vi "WSVCAP SHL FPGA LL Procedure I2C - Send Address Byte.vi"(0 "Procedure Step":T1, 1 "Wait Ticks Remaining":u32, 5 "I2C Wait Ticks":u32, 7 "Write Bits Remaining":u8, 9 "Write Byte":u8, 11 "error in (no error)":errorcluster, 13 "Socket Mask":u64 format="%012x", 14 "UUT Set (0/1)":u8) -> (3 "Wait Ticks Remaining Out":u32, 4 "Procedure Step Out":T1, 8 "Write Bits Remaining Out":u8, 10 "Finished":bool, 15 "error out":errorcluster)   [LabVIEW 2017]
uses:
  Type Defs/WSVCAP SHL Procedure Step Enum.ctl
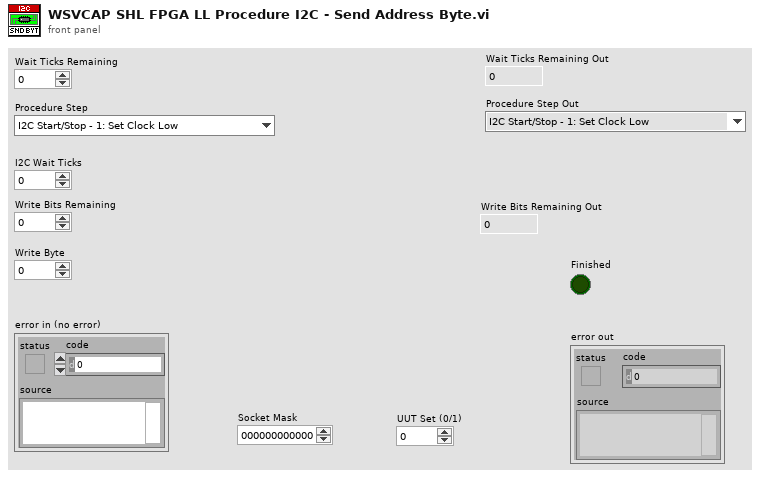
[diagram p1: front panel]
types:
  T1 = typedef "WSVCAP SHL Procedure Step Enum.ctl" = enum16{"I2C Start/Stop - 1: Set Clock Low", "I2C Start/Stop - 2: Wait", "I2C Start/Stop - 3: Set Data I", "I2C Start/Stop - 4: Wait", "I2C Start/Stop - 5: Set Clock High", "I2C Start/Stop - 6: Wait", "I2C Start/Stop - 7: Set Data II", "I2C Start/Stop - 8: Wait", "I2C Start/Stop - 9: Set Clock Low", "I2C Start/Stop - 10: Wait", "I2C Read ACK - 1: Set Clock High", "I2C Read ACK - 2: Wait", "I2C Read ACK - 3: Read ACK Bit", "I2C Read ACK - 4: Wait", "I2C Read ACK - 5: Set Clock Low", "I2C Read ACK - 6: Wait", "I2C Write ACK - 1: Write ACK Bit", "I2C Write ACK - 2: Wait", "I2C Write ACK - 3: Set Clock High", "I2C Write ACK - 4: Wait", "I2C Write ACK - 5: Set Clock Low", "I2C Write ACK - 6: Wait", "I2C Write ACK - 7: Set Data Low", "I2C Send Add - 1: Reset Bits Remaining", "I2C Send Add - 2: Set Data Bit", "I2C Send Add - 3: Wait", "I2C Send Add - 4: Set Clock High", "I2C Send Add - 5: Wait", "I2C Send Add - 6: Set Clock Low", "I2C Send Add - 7: Wait", "I2C Send Add - 8: Check Bits Remaining", "I2C Send Data - 1: Reset Bits Remaining", "I2C Send Data - 2: Load Write Bit from FIFO", "I2C Send Data - 3: Set Data Bit", "I2C Send Data - 4: Wait", "I2C Send Data - 5: Set Clock High", "I2C Send Data - 6: Wait", "I2C Send Data - 7: Set Clock Low", "I2C Send Data - 8: Wait", "I2C Send Data - 9: Check Bits Remaining", "I2C Receive Data - 1: Reset Bits Remaining", "I2C Receive Data - 2: Wait", "I2C Receive Data - 3: Set Clock High", "I2C Receive Data - 4: Wait", "I2C Receive Data - 5: Read Data Bit", "I2C Receive Data - 6: Wait", "I2C Receive Data - 7: Set Clock Low", "I2C Receive Data - 8: Wait", "I2C Receive Data - 9: Check Bits Remaining", "RFFE Send SSC - 1:Set Low", "RFFE Send SSC - 2:Wait", "RFFE Send SSC - 3:Set SDA High", "RFFE Send SSC - 4:Wait", "RFFE Send SSC - 5:Set SDA Low", "RFFE Send SSC - 6:Wait", "RFFE Send Data - 1:Set SCL High", "RFFE Send Data - 2:Wait", "RFFE Send Data - 3:Set SCL Low", "RFFE Send Data - 4:Wait", "RFFE Send Data - 5:Set SCL High (P)", "RFFE Send Data - 6:Wait", "RFFE Send Data - 7:Set SCL Low (P)", "RFFE Send Data - 8:Wait", "RFFE Send Data - 9:Set SCL High (BP)", "RFFE Send Data - 10:Wait", "RFFE Send Data - 11:Set SCL Low (BP)", "RFFE Send Data - 12:Wait", "RFFE Receive Data - 1:Set SCL High", "RFFE Receive Data - 2:Wait", "RFFE Receive Data - 3:Set SCL Low", "RFFE Receive Data - 4:Wait", "RFFE Receive Data - 5:Set SCL High (BP)", "RFFE Receive Data - 6:Wait", "RFFE Receive Data - 7:Set SCL Low (BP)", "RFFE Receive Data - 8:Wait", "RFFE Wait CMD Delay - 1:Wait", "RFFE Clear Lines - 1:Clear", "SRL Write Data - 1:Set SYNC High", "SRL Write Data - 2:Wait SYNC Delay", "SRL Write Data - 3:Set SYNC Low", "SRL Write Data - 4:Set SCLK High", "SRL Write Data - 5:Wait", "SRL Write Data - 6:Set SCLK Low", "SRL Write Data - 7:Wait", "SRL Write Data - 8:Set SYNC High", "SRL Wait CMD Delay - 1:Wait", "SRL Clear Lines - 1:Clear"}
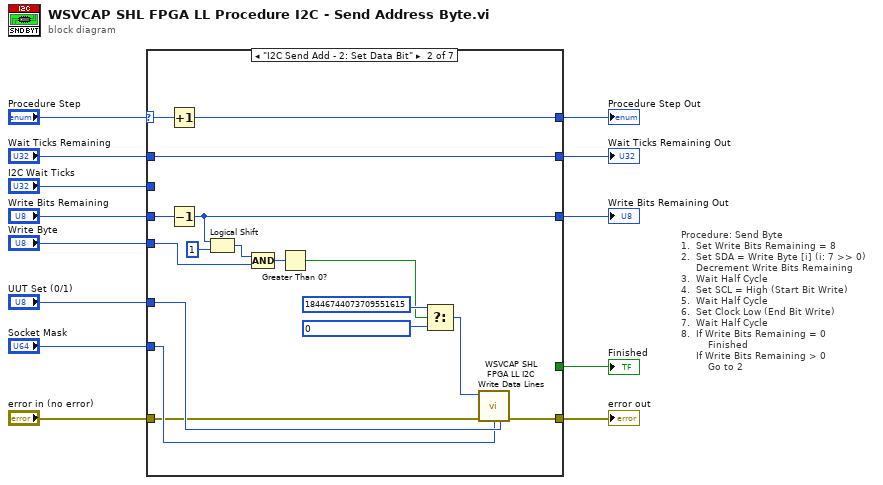
[diagram p0: block diagram]
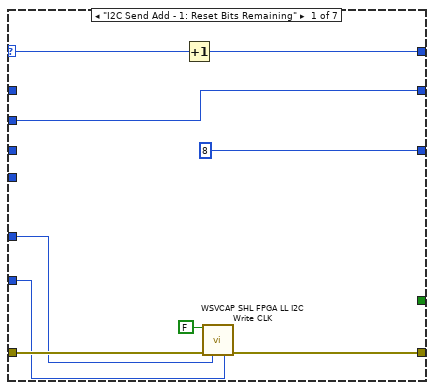
[diagram p2: hidden frame]
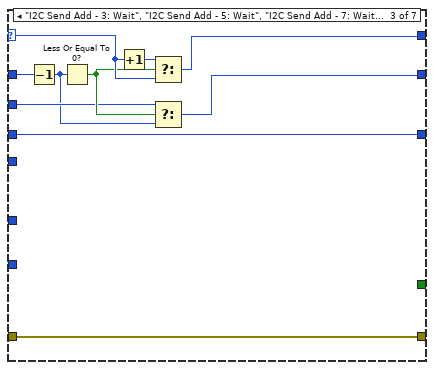
[diagram p3: hidden frame]
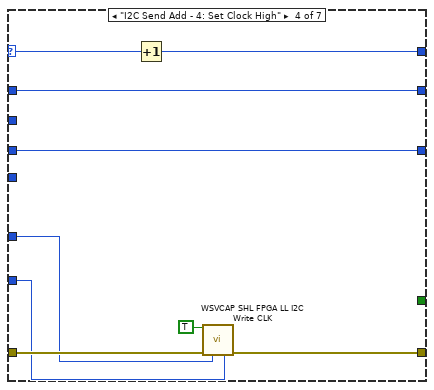
[diagram p4: hidden frame]
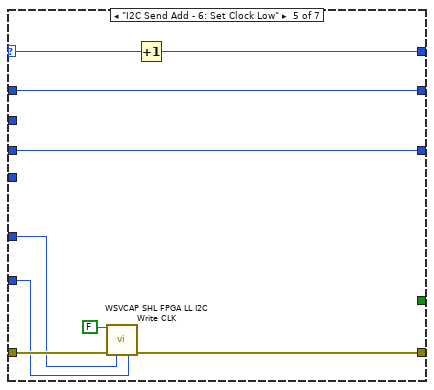
[diagram p5: hidden frame]
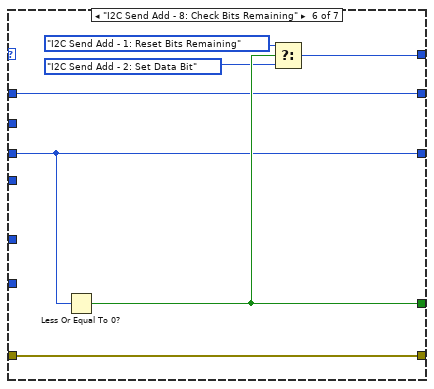
[diagram p6: hidden frame]
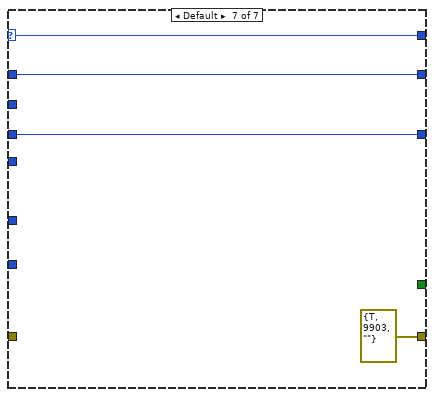
[diagram p7: hidden frame]
diagram:
  # "Procedure: Send Byte\n1.  Set Write Bits Remaining = 8\n2.  Set SDA = Write Byte [i] (i: 7 >> 0)\n     Decrement Write Bits Remaining\n3.  Wait Half Cycle\n4.  Set SCL = High (Start Bit Write)\n5.  Wait Half Cycle\n6.  Set Clock Low (End Bit Write)\n7.  Wait Half Cycle\n8.  If Write Bits Remaining = 0\n         Finished\n     If Write Bits Remaining > 0\n         Go to 2"
  n1 = case shown="\"I2C Send Add - 2: Set Data Bit\"" "Procedure Step" {
    selector: "Procedure Step" -> [w19 w39 w48 w56 w64 _ w77]
    tunnel: [w21 w23 w46 w57 w66 w74 errorcluster {"status"=TRUE, "code"=9903, "source"=""} ("error IO")] -> w12
    tunnel: "error in (no error)" -> [w22 w24 w46 w58 w67 w74 _]
    tunnel: "Wait Ticks Remaining" -> [_ w34 w49 w52 w61 w68 w76]
    tunnel: "I2C Wait Ticks" -> [w15 _ w44 _ _ _ _]
    tunnel: "Write Bits Remaining" -> [_ w37 w40 w51 w60 w69 w75]
    tunnel: "Write Byte" -> [_ w36 _ _ _ _ _]
    tunnel: [_ _ _ _ _ w73 _] -> w11
    tunnel: "Socket Mask" -> [w18 w25 _ w54 w63 _ _]
    tunnel: [w17 w35 w42 w53 w62 w70 w77] -> w4
    tunnel: [w15 w34 w41 w52 w61 w68 w76] -> w3
    tunnel: [u8 8 ("Write Bits Remaining") w33 w40 w51 w60 w69 w75] -> w2
    tunnel: "UUT Set (0/1)" -> [w14 w26 _ w50 w59 _ _]
    frame "I2C Send Add - 1: Reset Bits Remaining" {
      n2 = Increment(x=w19) -> (x+1=w17:T1)
      n3 = call "WSVCAP SHL FPGA LL I2C Write CLK.vi"("Bit In"=FALSE, "error in (no error)"=w22, "UUT Set (0/1 (Legacy)"=w14, "Socket Mask"=w18) -> ("error out"=w21:errorcluster)  [unwired: 11 in]
    }
    frame "I2C Send Add - 2: Set Data Bit" {
      n4 = Increment(x=w39) -> (x+1=w35:T1)
      n5 = Decrement(x=w37) -> (x-1=w33:u8)
      n6 = Logical Shift(y=w33, x=u8 1) -> (x << y=w31:u8)
      n7 = Compound Arithmetic op=AND(w31, w36) -> (w38:u8)
      n8 = Greater Than 0?(x=w38) -> (x > 0?=w27:bool)
      n9 = Select(t=u64 18446744073709551615 ("Write Bit (U64)"), s=w27, f=u64 0 ("Write Bit (U64)")) -> (s? t:f=w28:u64)
      n10 = call "WSVCAP SHL FPGA LL I2C Write Data Lines.vi"("Write Bit (U64)"=w28, "error in (no error)"=w24, "Socket Mask"=w25, "UUT Set (0/1) (Legacy)"=w26) -> ("error out"=w23:errorcluster)  [unwired: 11 in]
    }
    frame "I2C Send Add - 3: Wait", "I2C Send Add - 5: Wait", "I2C Send Add - 7: Wait" {
      n11 = Decrement(x=w49) -> (x-1=w43:u32)
      n12 = Less Or Equal To 0?(x=w43) -> (x <= 0?=w45:bool)
      n13 = Increment(x=w48) -> (x+1=w47:T1)
      n14 = Select(t=w47, s=w45, f=w48) -> (s? t:f=w42:T1)
      n15 = Select(t=w44, s=w45, f=w43) -> (s? t:f=w41:u32)
    }
    frame "I2C Send Add - 4: Set Clock High" {
      n16 = Increment(x=w56) -> (x+1=w53:T1)
      n17 = call "WSVCAP SHL FPGA LL I2C Write CLK.vi"("Bit In"=TRUE, "error in (no error)"=w58, "UUT Set (0/1 (Legacy)"=w50, "Socket Mask"=w54) -> ("error out"=w57:errorcluster)  [unwired: 11 in]
    }
    frame "I2C Send Add - 6: Set Clock Low" {
      n18 = call "WSVCAP SHL FPGA LL I2C Write CLK.vi"("Bit In"=FALSE, "error in (no error)"=w67, "UUT Set (0/1 (Legacy)"=w59, "Socket Mask"=w63) -> ("error out"=w66:errorcluster)  [unwired: 11 in]
      n19 = Increment(x=w64) -> (x+1=w62:T1)
    }
    frame "I2C Send Add - 8: Check Bits Remaining" {
      n20 = Less Or Equal To 0?(x=w69) -> (x <= 0?=w73:bool)
      n21 = Select(t=WSVCAP_SHL_Procedure_Step_Enum."I2C Send Add - 1: Reset Bits Remaining" ("Procedure Step"), s=w73, f=WSVCAP_SHL_Procedure_Step_Enum."I2C Send Add - 2: Set Data Bit" ("Procedure Step")) -> (s? t:f=w70:T1)
    }
    frame Default {
    }
  }
  "error out" <- w12
  "Finished" <- w11
  "Procedure Step Out" <- w4
  "Wait Ticks Remaining Out" <- w3
  "Write Bits Remaining Out" <- w2
